vi "Data_Packet_Test.vi"() -> ()   [LabVIEW 2017]
uses:
  Controls/Data Packets/Data_Packet.ctl
  Controls/Packet/Packet.ctl
  Controls/Packet/Packet_Direction.ctl
  Controls/Packet/Packet_Type.ctl
  Controls/Packet/Packet_Priority.ctl
  Controls/Data Packets/Parameter.ctl
  Controls/Data Packets/Parameter_Data_Type.ctl
  Controls/Data Packets/Data_Packet_FGV_Commands.ctl
panel:
  out "Parameter value out":string
  out "Data Packets Out":T1[](array[typedef])
  in  "Parameter value in":string
  in  "Parameter name":string
  out "Parameter names":string[](array[string])
  in  "Symbol File Path":path
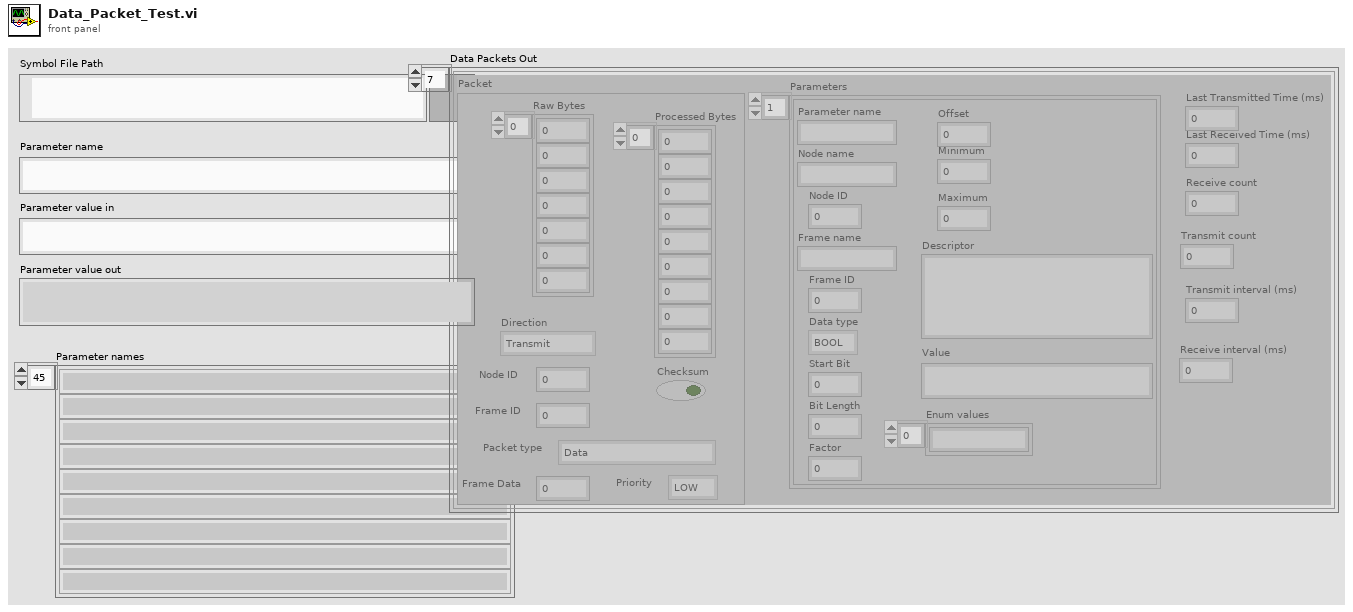
[diagram p1: front panel]
types:
  T1 = typedef "Data_Packet.ctl" = cluster{"Packet":T2, "Parameters":T6[], "Last Received Time (ms)":u64, "Receive count":u32, "Transmit count":u32, "Transmit interval (ms)":u32, "Last Transmitted Time (ms)":u64, "Receive interval (ms)":u32}
  T2 = typedef "Packet.ctl" = cluster{"Raw Bytes":u8[], "Checksum":bool, "Direction":T3, "Processed Bytes":u8[], "Node ID":u8, "Packet type":T4, "Frame Data":u32, "Priority":T5, "Frame ID":u8}
  T3 = typedef "Packet_Direction.ctl" = enum16{"Transmit", "Receive", "Bidirectional"}
  T4 = typedef "Packet_Type.ctl" = enum16{"Data", "Connection Management", "Remote Request", "Error/Status"}
  T5 = typedef "Packet_Priority.ctl" = enum16{"LOW", "HIGH"}
  T6 = typedef "Parameter.ctl" = cluster{"Parameter name":string, "Node name":string, "Node ID":u8, "Frame name":string, "Frame ID":u8, "Data type":T7, "Start Bit":i32, "Bit Length":i32, "Factor":dbl, "Offset":dbl, "Minimum":dbl, "Maximum":dbl, "Descriptor":string, "Enum values":string[], "Value":string}
  T7 = typedef "Parameter_Data_Type.ctl" = enum16{"BOOL", "UNSIGNED", "SIGNED", "FLOAT32", "ENUM"}
  T8 = typedef "Data_Packet_FGV_Commands.ctl" = enum16{"Update all parameters from data packets", "Update Packet", "Load", "Read Packet Parameters", "Write Packet Parameters", "Read Packet Parameter", "Write Packet Parameter", "Read Data Packets", "Read Data Packet", "Read Data Packet by Parameter Name", "Get Parameter Node and Frame ID", "Read Data Packet from Node ID and Frame ID"}
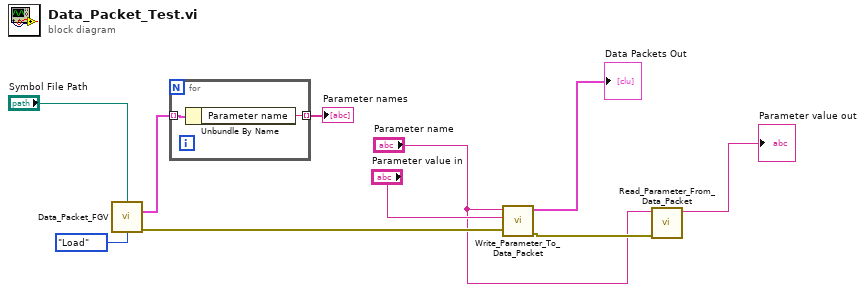
[diagram p0: block diagram]
diagram:
  n1 = call "Data_Packet_FGV.vi"("Symbol File Path"="Symbol File Path", "Commands"=Data_Packet_FGV_Commands."Load") -> ("Parameters out"=w8:T6[], "error out"=w9:errorcluster)  [unwired: 8 in, 4 out]
  n2 = for {
    tunnel: w8 -> [w12] mode=indexing
    tunnel: [w11] -> w7 mode=indexing
    n3 = Unbundle By Name(w12) -> ("Parameter name"=w11:string)
  }
  "Parameter names" <- w7
  n4 = call "Write_Parameter_To_Data_Packet.vi"("error in (no error)"=w9, "Parameter value"="Parameter value in", "Parameter name"="Parameter name") -> ("error out"=w3:errorcluster, "Data Packets Out"=→"Data Packets Out":T1[])  [unwired: 7 in]
  n5 = call "Read_Parameter_From_Data_Packet.vi"("error in (no error)"=w3, "Parameter name"="Parameter name") -> ("Parameter value out"=→"Parameter value out":string)  [unwired: 8 in, 1 out]
